vi "moreSamplesToPlayback.vi"(0 "Device":i32, 1 "playbackCycleLength":i32, 2 "previousSampleCycle":i32) -> (7 "ReadyForMore":bool, 10 "currentSampleCycle":i32)   [LabVIEW 2011]
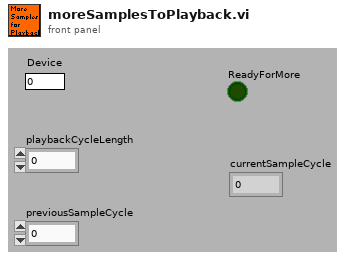
[diagram p1: front panel]
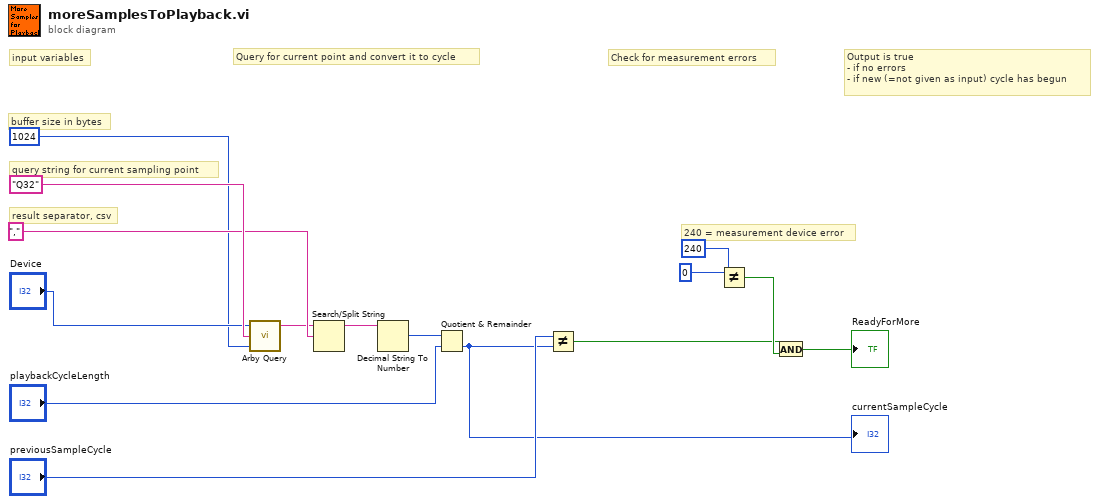
[diagram p0: block diagram]
diagram:
  # "Output is true\n- if no errors\n- if new (=not given as input) cycle has begun"
  # "Check for measurement errors"
  # "Query for current point and convert it to cycle"
  # "input variables"
  # "result separator, csv"
  # "240 = measurement device error"
  # "query string for current sampling point"
  # "buffer size in bytes"
  n1 = call "Arby Query.vi"("Reply size"=1024, "Query"="Q32", "Device"="Device") -> ("Reply"=w11:string)  [unwired: 2 out]
  n2 = Search/Split String(string=w11, search string/char (-)=",") -> (substring before match=w13:string)  [unwired: 1 in, 2 out]
  n3 = Decimal String To Number(string=w13) -> (number=w12:i32)  [unwired: 2 in, 1 out]
  n4 = Quotient & Remainder(x=w12, y="playbackCycleLength") -> (floor(x/y)=w1:i32)  [unwired: 1 out]
  "currentSampleCycle" <- w1
  n5 = Not Equal?(x="previousSampleCycle", y=w1) -> (x != y?=w3:bool)
  n6 = Not Equal?(x=0, y=240) -> (x != y?=w7:bool)
  n7 = And(x=w3, y=w7) -> (x .and. y?=→"ReadyForMore":bool)
